vi "Drop Sand (Floor).vi"(5 "Y in":i32, 6 "Floor-1":i32, 7 "X in":i32, 8 "Bottom in":i32[](array[numeric]), 9 "Top in":i32[](array[numeric]), 10 "Right in":i32[](array[numeric]), 11 "Left in":i32[](array[numeric])) -> (0 "Bottom out":i32[](array[numeric]), 1 "Top out":i32[](array[numeric]), 2 "Right out":i32[](array[numeric]), 3 "Left out":i32[](array[numeric]), 4 "Filled?":bool)   [LabVIEW 2021, in "d14.lvlib"]
uses:
  d14.lvlib
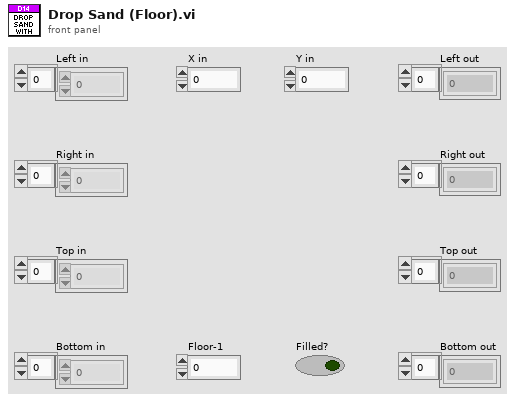
[diagram p1: front panel]
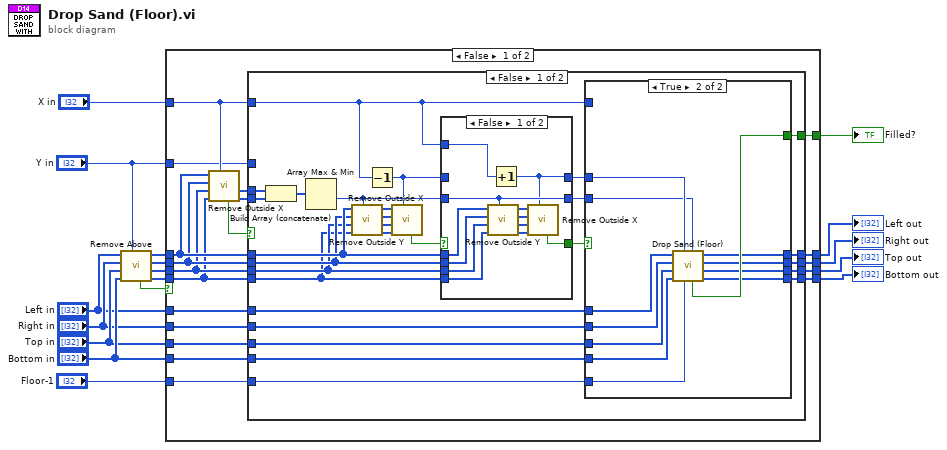
[diagram p0: block diagram]
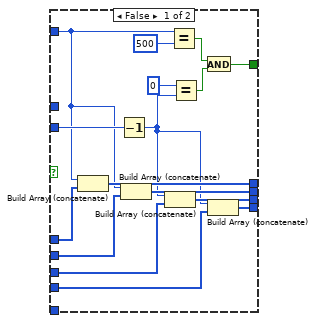
[diagram p2: hidden frame]
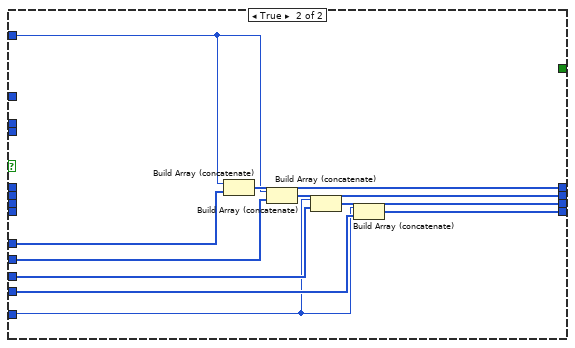
[diagram p4: hidden frame]
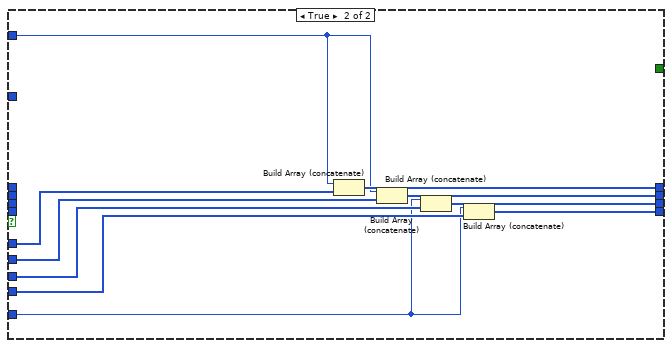
[diagram p5: hidden frame]
diagram:
  n1 = call "Remove Above.vi"("Y in"="Y in", "Bottom in"="Bottom in", "Top in"="Top in", "Right in"="Right in", "Left in"="Left in") -> ("Bottom out"=w13:i32[], "Top out"=w14:i32[], "Right out"=w15:i32[], "Left out"=w16:i32[], "empty?"=w10:bool)  [unwired: 2 in]
  n2 = case shown="False" w10 {
    tunnel: "X in" -> [w36 w122]
    tunnel: w16 -> [w35 _]
    tunnel: w15 -> [w34 _]
    tunnel: w14 -> [w33 _]
    tunnel: w13 -> [w32 _]
    tunnel: "Y in" -> [w31 _]
    tunnel: [w30 _] -> w11
    tunnel: [w26 w123] -> w9
    tunnel: [w25 w120] -> w8
    tunnel: [w24 w118] -> w6
    tunnel: [w23 w119] -> w7
    tunnel: "Bottom in" -> [w22 w124]
    tunnel: "Top in" -> [w21 w125]
    tunnel: "Right in" -> [w20 w126]
    tunnel: "Left in" -> [w19 w127]
    tunnel: "Floor-1" -> [w18 w121]
    frame False {
      n3 = call "Remove Outside X.vi"("X in"=w36, "Bottom in"=w32, "Top in"=w33, "Right in"=w34, "Left in"=w35) -> ("Bottom out"=w28:i32[], "Top out"=w29:i32[], "empty?"=w27:bool)  [unwired: 2 in, 2 out]
      n4 = case shown="False" w27 {
        tunnel: w36 -> [w42 w112]
        tunnel: w35 -> [w56 _]
        tunnel: w34 -> [w55 _]
        tunnel: w33 -> [w54 _]
        tunnel: w32 -> [w53 _]
        tunnel: w31 -> [_ _]
        tunnel: [w49 _] -> w30
        tunnel: w29 -> [w60 _]
        tunnel: w28 -> [w59 _]
        tunnel: [w48 w117] -> w26
        tunnel: [w47 w108] -> w25
        tunnel: [w46 w109] -> w23
        tunnel: [w45 w110] -> w24
        tunnel: w22 -> [w41 w113]
        tunnel: w21 -> [w40 w114]
        tunnel: w20 -> [w39 w115]
        tunnel: w19 -> [w38 w116]
        tunnel: w18 -> [w37 w111]
        frame False {
          n5 = Build Array (concatenate)(w60, w59) -> (w58:i32[])
          n6 = Array Max & Min(array=w58) -> (min value=w52:i32)  [unwired: 3 out]
          n7 = call "Remove Outside Y.vi"("Y in"=w52, "Bottom in"=w53, "Top in"=w54, "Right in"=w55, "Left in"=w56) -> ("Bottom out"=w64:i32[], "Top out"=w63:i32[], "Right out"=w62:i32[], "Left out"=w61:i32[])  [unwired: 2 in, 1 out]
          n8 = Decrement(x=w42) -> (x-1=w44:i32)
          n9 = call "Remove Outside X.vi"("X in"=w44, "Bottom in"=w64, "Top in"=w63, "Right in"=w62, "Left in"=w61) -> ("empty?"=w57:bool)  [unwired: 2 in, 4 out]
          n10 = case shown="False" w57 {
            selector: w57 -> [_ w107]
            tunnel: w56 -> [w98 _]
            tunnel: w55 -> [w97 _]
            tunnel: w54 -> [w96 _]
            tunnel: w53 -> [w95 _]
            tunnel: w42 -> [w100 _]
            tunnel: w52 -> [w94 w106]
            tunnel: [w99 w107] -> w51
            tunnel: [w94 w106] -> w50
            tunnel: w44 -> [_ w105]
            tunnel: [w93 w105] -> w43
            frame False {
              n11 = call "Remove Outside Y.vi"("Y in"=w94, "Bottom in"=w95, "Top in"=w96, "Right in"=w97, "Left in"=w98) -> ("Bottom out"=w101:i32[], "Top out"=w104:i32[], "Right out"=w103:i32[], "Left out"=w102:i32[])  [unwired: 2 in, 1 out]
              n12 = Increment(x=w100) -> (x+1=w93:i32)
              n13 = call "Remove Outside X.vi"("X in"=w93, "Bottom in"=w101, "Top in"=w104, "Right in"=w103, "Left in"=w102) -> ("empty?"=w99:bool)  [unwired: 2 in, 4 out]
            }
            frame True {
            }
          }
          n14 = case shown="True" w51 {
            tunnel: w43 -> [_ w92]
            tunnel: w50 -> [w76 w91]
            tunnel: [w65 w90] -> w49
            tunnel: [w80 w89] -> w48
            tunnel: [w79 w88] -> w47
            tunnel: [w78 w87] -> w46
            tunnel: [w77 w86] -> w45
            tunnel: w42 -> [w69 _]
            tunnel: w41 -> [w75 w82]
            tunnel: w40 -> [w74 w83]
            tunnel: w39 -> [w73 w84]
            tunnel: w38 -> [w72 w85]
            tunnel: w37 -> [_ w81]
            frame False {
              n15 = Build Array (concatenate)(w69, w72) -> (w80:i32[])
              n16 = Decrement(x=w76) -> (x-1=w71:i32)
              n17 = Build Array (concatenate)(w69, w73) -> (w79:i32[])
              n18 = Build Array (concatenate)(w71, w74) -> (w78:i32[])
              n19 = Equal?(x=w69, y=500) -> (x = y?=w67:bool)
              n20 = Equal?(x=0, y=w71) -> (x = y?=w66:bool)
              n21 = And(x=w67, y=w66) -> (x .and. y?=w65:bool)
              n22 = Build Array (concatenate)(w71, w75) -> (w77:i32[])
            }
            frame True {
              n23 = call "Drop Sand (Floor).vi"("Y in"=w91, "Floor-1"=w81, "X in"=w92, "Bottom in"=w82, "Top in"=w83, "Right in"=w84, "Left in"=w85) -> ("Bottom out"=w86:i32[], "Top out"=w87:i32[], "Right out"=w88:i32[], "Left out"=w89:i32[], "Filled?"=w90:bool)
            }
          }
        }
        frame True {
          n24 = Build Array (concatenate)(w112, w116) -> (w117:i32[])
          n25 = Build Array (concatenate)(w112, w115) -> (w108:i32[])
          n26 = Build Array (concatenate)(w111, w114) -> (w109:i32[])
          n27 = Build Array (concatenate)(w111, w113) -> (w110:i32[])
        }
      }
    }
    frame True {
      n28 = Build Array (concatenate)(w122, w127) -> (w123:i32[])
      n29 = Build Array (concatenate)(w122, w126) -> (w120:i32[])
      n30 = Build Array (concatenate)(w121, w125) -> (w119:i32[])
      n31 = Build Array (concatenate)(w121, w124) -> (w118:i32[])
    }
  }
  "Filled?" <- w11
  "Left out" <- w9
  "Right out" <- w8
  "Top out" <- w7
  "Bottom out" <- w6
